vi "COMI INT Stop.vi"(11 "hDevice":u32) -> (2 "function return":i32, 3 "hDevice out":u32)   [LabVIEW 2017, in "Comidll.lvlib"]
doc: "long (COMI_INT_Stop) (HANDLE hDevice);"
uses:
  <userlib>/Comidll/Comidll.lvlib
  <userlib>/Comidll/Comidll.dll
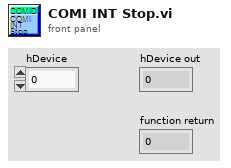
[diagram p1: front panel]
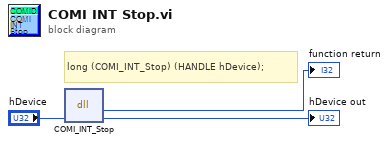
[diagram p0: block diagram]
diagram:
  # "long\t(COMI_INT_Stop) (HANDLE hDevice);"
  n1 = dll-call lib="C:/Program Files/National Instruments/LabVIEW 2017/user.lib/Comidll/Comidll.*" fn="COMI_INT_Stop"("hDevice"="hDevice") -> (→"function return":i32, "hDevice"=→"hDevice out":u32)  [unwired: 3 in, 2 out]
